vi "Init.vi"(8 "error in":errorcluster, 11 "DAQmx Base CFG in":refnum<class "DAQmx Base CFG.lvclass">) -> (0 "error out":errorcluster, 3 "DAQmx Base CFG out":refnum<class "DAQmx Base CFG.lvclass">)   [LabVIEW 2023, in "DAQmx Base CFG.lvclass"]
uses:
  DAQmx Base CFG.lvclass
  DAQmx Base CFG.lvclass/DAQmx Base CFG.ctl
  Configurations/CFG JSON/CFG JSON.lvclass
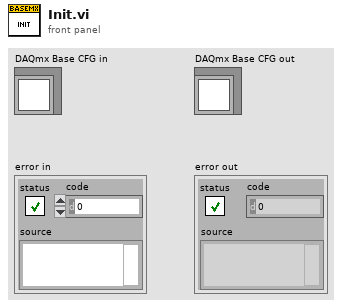
[diagram p1: front panel]
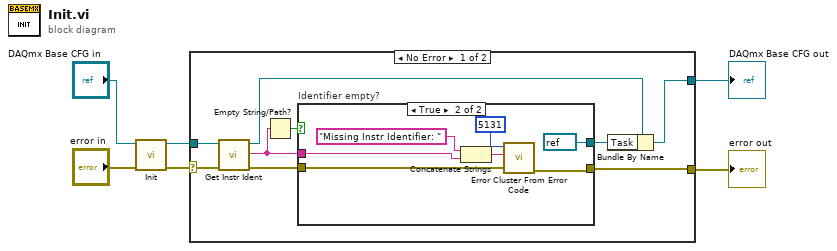
[diagram p0: block diagram]
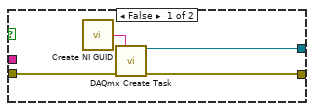
[diagram p2: hidden frame]
diagram:
  n1 = call-parent "Init.vi"("error in"="error in", "CFG Base in"="DAQmx Base CFG in") -> ("error out"=w3:errorcluster, "CFG Base out"=w1:refnum<class "DAQmx Base CFG.lvclass">)  [unwired: 8 in]
  n2 = case shown="No Error" w3 {
    selector: w3 -> [w15 w27]
    tunnel: w1 -> [w14 w28]
    tunnel: [w9 w28] -> w5
    tunnel: [w11 w27] -> w4
    frame No Error {
      n3 = call-dynamic "Get Instr Ident.vi"("error in"=w15, "CFG JSON in"=w14) -> ("error out"=w12:errorcluster, "Instr Ident"=w7:string, "CFG JSON out"=w10:refnum<class "DAQmx Base CFG.lvclass">)  [unwired: 7 in]
      n4 = Empty String/Path?(string/path=w7) -> (empty?=w13:bool)
      n5 = case "Identifier empty?" shown="True" w13 {
        tunnel: w12 -> [w19 w25]
        tunnel: [w18 w24] -> w11
        tunnel: [w16 refnum<k21> refnum ("task out")] -> w8
        tunnel: w7 -> [_ w20]
        frame False {
          n6 = call <vilib>:"Create NI GUID.vi"() -> ("NI GUID"=w17:string)
          n7 = call <vilib>:"DAQmx Create Task.vi"("new task name"=w17, "error in"=w19) -> ("task out"=w16:refnum<k21>, "error out"=w18:errorcluster)  [unwired: 12 in]
        }
        frame True {
          n8 = Concatenate Strings("Missing Instr Identifier: ", w20) -> (w22:string)
          n9 = call <vilib>:"Error Cluster From Error Code.vi"("error in (no error)"=w25, "error message (\"\")"=w22, "error code (0)"=5131) -> ("error out"=w24:errorcluster)  [unwired: 6 in]
        }
      }
      n10 = Bundle By Name(cluster=w10, "Task"=w8) -> (w9:refnum<class "DAQmx Base CFG.lvclass">)
    }
    frame Error {
    }
  }
  "error out" <- w4
  "DAQmx Base CFG out" <- w5
